vi "TCL Baseline Match.vi"(2 "Fragments Desired":string[](array[string]), 3 "Fragments to Match":T1(array[cluster])) -> (0 "Event Data":string[][](array[string]), 1 "Fragments Returned":string[](array[string]))   [LabVIEW 2009]
doc: "This VI goes through some painful manipulations to provide what in a SQL-based system would take one SELECT statement. The user provides match criteria in Fragments to Match, and in Event Data gets back (for all matching events) all available items from that were specified in Fragments Desired."
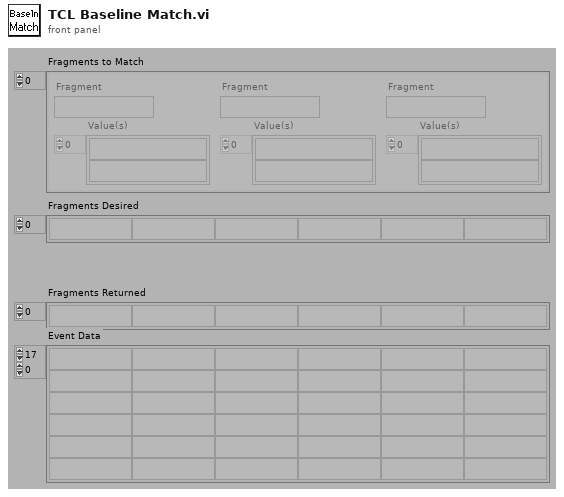
[diagram p1: front panel]
types:
  T1 = cluster{"Fragment":string, "Value(s)":string[]}[]
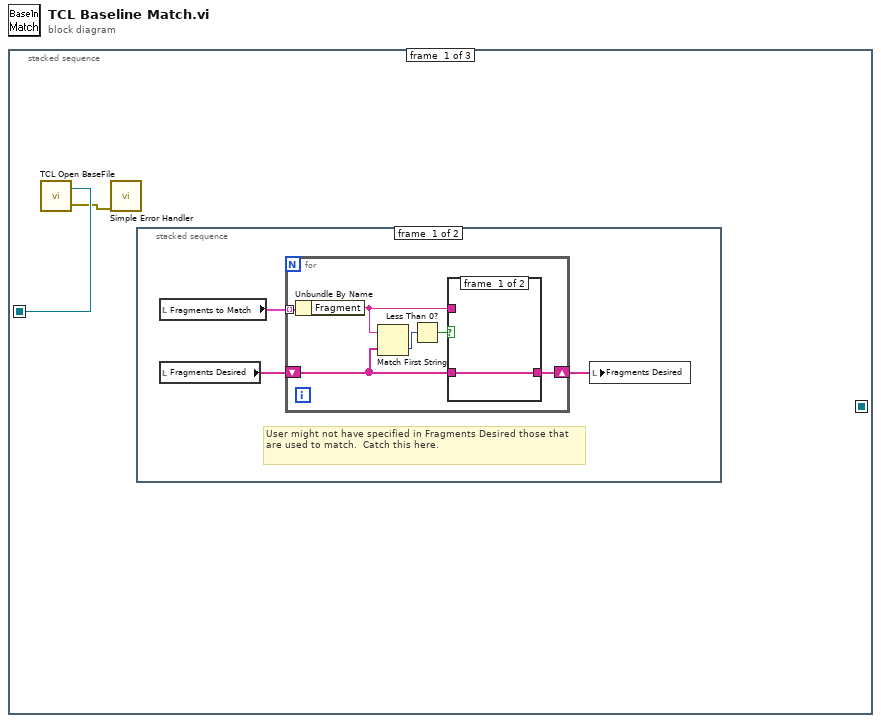
[diagram p0: block diagram]
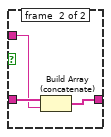
[diagram p2: hidden frame]
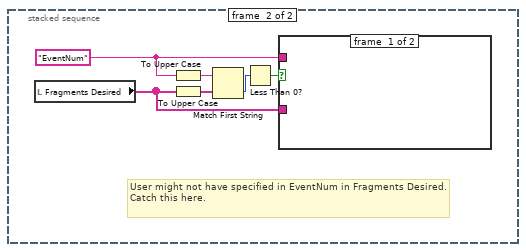
[diagram p3: hidden frame]
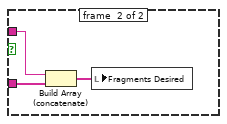
[diagram p4: hidden frame]
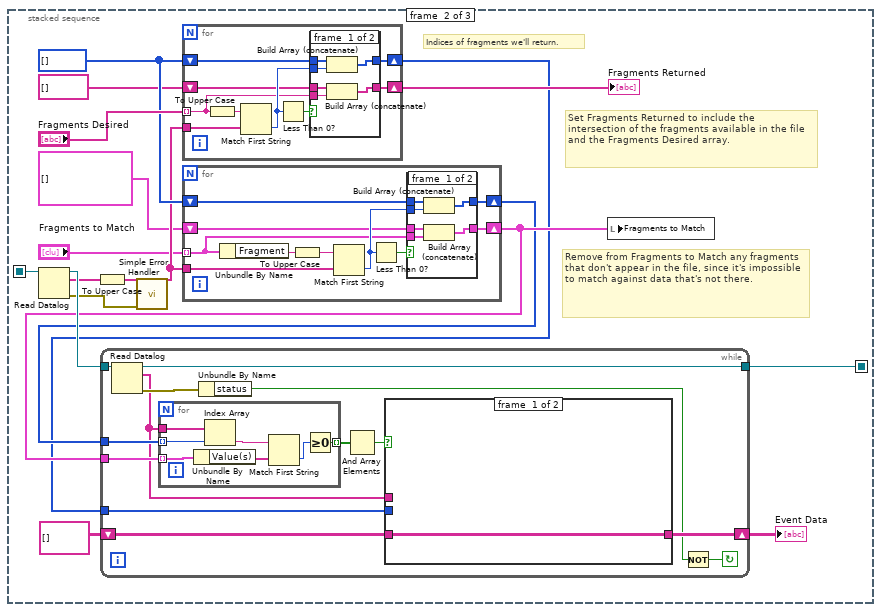
[diagram p5: hidden frame]
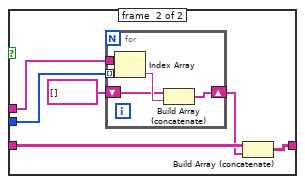
[diagram p6: hidden frame]
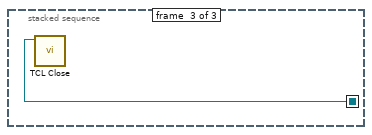
[diagram p9: hidden frame]
diagram:
  n1 = stacked-sequence {
    seq-local: [w2 _ _] -> [_ w40 _]
    seq-local: [_ w37 _] -> [_ _ w109]
    frame #0 {
      n2 = call "TCL Open BaseFile.vi"() -> ("error out"=w1:errorcluster, "Event File Refnum"=w2:refnum<k1>)
      n3 = call <vilib>:"Simple Error Handler.vi"("error in (no error)"=w1) -> ()  [unwired: 4 in, 5 out]
      n4 = stacked-sequence {
        frame #0 {
          # "User might not have specified in Fragments Desired those that are used to match.  Catch this here."
          n5 = local read "Fragments to Match"() -> (w5:T1)
          n6 = local read "Fragments Desired"() -> (w4:string[])
          n7 = for {
            tunnel: w5 -> [w11] mode=indexing
            shift-right: [w7] -> w3
            shift-left: w4 -> [w8]
            n8 = Unbundle By Name(w11) -> ("Fragment"=w6:string)
            n9 = Match First String(2:w8, 3:w6) -> (0:w10:i32)  [unwired: 1 out]
            n10 = Less Than 0?(x=w10) -> (x < 0?=w9:bool)
            n11 = case shown="True" w9 {
              tunnel: [w12 w14] -> w7
              tunnel: w8 -> [w12 w15]
              tunnel: w6 -> [_ w13]
              frame #0 {
              }
              frame #1 {
                n12 = Build Array (concatenate)(w15, w13) -> (w14:string[])
              }
            }
          }
          n13 = local write "Fragments Desired"(w3) -> ()
        }
        frame #1 {
          w20 = "EventNum"
          # "User might not have specified in EventNum in Fragments Desired.  Catch this here."
          n14 = local read "Fragments Desired"() -> (w21:string[])
          n15 = To Upper Case(1:w20) -> (0:w16:string)
          n16 = To Upper Case(1:w21) -> (0:w17:string[])
          n17 = Match First String(2:w17, 3:w16) -> (0:w18:i32)  [unwired: 1 out]
          n18 = Less Than 0?(x=w18) -> (x < 0?=w19:bool)
          n19 = case shown="True" w19 {
            tunnel: w20 -> [_ w24]
            tunnel: w21 -> [_ w23]
            frame #0 {
            }
            frame #1 {
              n20 = Build Array (concatenate)(w24, w23) -> (w22:string[])
              n21 = local write "Fragments Desired"(w22) -> ()
            }
          }
        }
      }
    }
    frame #1 {
      w34 = i32[] []
      # "Indices of fragments we'll return."
      # "Set Fragments Returned to include the intersection of the fragments available in the file and the Fragments Desired array."
      # "Remove from Fragments to Match any fragments that don't appear in the file, since it's impossible to match against data that's not there."
      n22 = Read Datalog(7:w40) -> (0:w25:errorcluster, 2:w26:string[], 3:w39:refnum<k1>)  [unwired: 2 in]
      n23 = To Upper Case(1:w26) -> (0:w33:string[])
      n24 = call <vilib>:"Simple Error Handler.vi"("error in (no error)"=w25) -> ()  [unwired: 4 in, 5 out]
      n25 = for {
        tunnel: w33 -> [w100]
        tunnel: "Fragments Desired" -> [w93] mode=indexing
        shift-right: [w96] -> w27
        shift-left: w34 -> [w97]
        shift-right: [w94] -> w41
        shift-left: string[] [] -> [w95]
        n26 = To Upper Case(1:w93) -> (0:w92:string)
        n27 = Match First String(2:w100, 3:w92) -> (0:w99:i32)  [unwired: 1 out]
        n28 = Less Than 0?(x=w99) -> (x < 0?=w98:bool)
        n29 = case shown="False" w98 {
          tunnel: w99 -> [w101 _]
          tunnel: w97 -> [w106 w108]
          tunnel: [w105 w108] -> w96
          tunnel: w95 -> [w104 w107]
          tunnel: [w103 w107] -> w94
          tunnel: w93 -> [w102 _]
          frame #0 {
            n30 = Build Array (concatenate)(w106, w101) -> (w105:i32[])
            n31 = Build Array (concatenate)(w104, w102) -> (w103:string[])
          }
          frame #1 {
          }
        }
      }
      "Fragments Returned" <- w41
      n32 = for {
        tunnel: w33 -> [w83]
        tunnel: "Fragments to Match" -> [w75] mode=indexing
        shift-right: [w79] -> w28
        shift-left: w34 -> [w80]
        shift-right: [w77] -> w30
        shift-left: T1 [] ("Fragments to Match") -> [w78]
        n33 = Unbundle By Name(w75) -> ("Fragment"=w74:string)
        n34 = To Upper Case(1:w74) -> (0:w76:string)
        n35 = Match First String(2:w83, 3:w76) -> (0:w82:i32)  [unwired: 1 out]
        n36 = Less Than 0?(x=w82) -> (x < 0?=w81:bool)
        n37 = case shown="False" w81 {
          tunnel: w82 -> [w84 _]
          tunnel: w80 -> [w89 w91]
          tunnel: [w88 w91] -> w79
          tunnel: w78 -> [w87 w90]
          tunnel: [w86 w90] -> w77
          tunnel: w75 -> [w85 _]
          frame #0 {
            n38 = Build Array (concatenate)(w89, w84) -> (w88:i32[])
            n39 = Build Array (concatenate)(w87, w85) -> (w86:T1)
          }
          frame #1 {
          }
        }
      }
      n40 = while {
        tunnel: w27 -> [w47]
        tunnel: w28 -> [w49]
        tunnel: w30 -> [w50]
        shift-left: string[][] [] ("Data") -> [w52]
        shift-right: [w51] -> w36
        tunnel: [w53] -> w37
        tunnel: w39 -> [w54]
        stop <- w44 continue-if-true
        n41 = Read Datalog(7:w54) -> (0:w45:errorcluster, 2:w43:string[], 3:w53:refnum<k1>)  [unwired: 2 in]
        n42 = for {
          tunnel: w50 -> [w61] mode=indexing
          tunnel: w43 -> [w60]
          tunnel: w49 -> [w59] mode=indexing
          tunnel: [w55] -> w48 mode=indexing
          n43 = Unbundle By Name(w61) -> ("Value(s)"=w58:string[])
          n44 = Index Array(array=w60, index=w59) -> (element=w57:string)
          n45 = Match First String(2:w58, 3:w57) -> (0:w56:i32)  [unwired: 1 out]
          n46 = Greater Or Equal To 0?(x=w56) -> (x >= 0?=w55:bool)
        }
        n47 = Unbundle By Name(w45) -> ("status"=w42:bool)
        n48 = And Array Elements(Boolean array=w48) -> (logical AND=w46:bool)
        n49 = case shown="True" w46 {
          tunnel: w43 -> [_ w67]
          tunnel: w47 -> [_ w68]
          tunnel: w52 -> [w62 w66]
          tunnel: [w62 w65] -> w51
          frame #0 {
          }
          frame #1 {
            n50 = for {
              tunnel: w68 -> [w72] mode=indexing
              tunnel: w67 -> [w73]
              shift-right: [w69] -> w64
              shift-left: string[] [] -> [w70]
              n51 = Index Array(array=w73, index=w72) -> (element=w71:string)
              n52 = Build Array (concatenate)(w70, w71) -> (w69:string[])
            }
            n53 = Build Array (concatenate)(w66, w64) -> (w65:string[][])
          }
        }
        n54 = Not(x=w42) -> (.not. x?=w44:bool)
      }
      "Event Data" <- w36
      n55 = local write "Fragments to Match"(w30) -> ()
    }
    frame #2 {
      n56 = call "TCL Close.vi"("Event File Refnum"=w109) -> ()  [unwired: 3 in]
    }
  }
